vi "FilePaths.vi"(8 "error in":errorcluster) -> (0 "error out":errorcluster, 2 "paths":T1)   [LabVIEW 2013, in "Advanced Configuration Tool.lvlib"]
doc: "This VI has the Path to the Classes and the Glyphs, Additional Behavior might be added if you want to load them from a different path. By default they are in Glyphs folder and Classes folder in the main directory"
uses:
  Advanced Configuration Tool.lvlib
  Controls/FilePaths.ctl
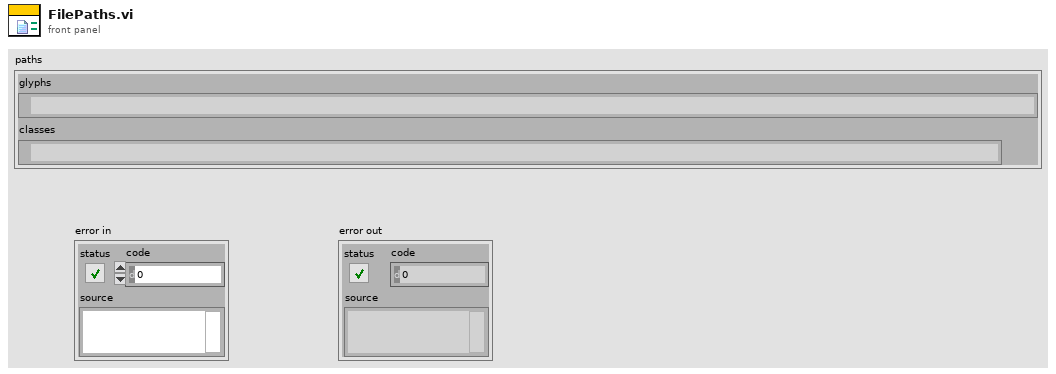
[diagram p1: front panel]
types:
  T1 = typedef "Advanced Configuration Tool.lvlib/FilePaths.ctl" = cluster{"glyphs":path, "classes":path}
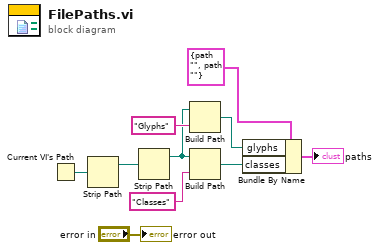
[diagram p0: block diagram]
diagram:
  n1 = Current VI's Path() -> (path=w3:path)
  n2 = Strip Path(path=w3) -> (stripped path=w1:path)  [unwired: 1 out]
  n3 = Strip Path(path=w1) -> (stripped path=w2:path)  [unwired: 1 out]
  n4 = Build Path(base path=w2, name or relative path="Glyphs") -> (appended path=w7:path)
  n5 = Build Path(base path=w2, name or relative path="Classes") -> (appended path=w4:path)
  n6 = Bundle By Name(cluster=T1 {"glyphs"=path "", "classes"=path ""} ("Cluster 2"), "glyphs"=w7, "classes"=w4) -> (→"paths":T1)
  "error out" <- "error in"
